vi "IV_Sweep.vi"(8 "error in":errorcluster, 11 "Transport":refnum<class "Transport.lvclass">) -> (0 "error out":errorcluster, 3 "Transport out":refnum<class "Transport.lvclass">)   [LabVIEW 2016, in "Transport.lvclass"]
uses:
  Transport.lvclass
  Control Experiment/Typedefs/Instruments--cluster.ctl
  <userlib>/LevyLab/Krohn Hite 7008/Instrument.KH7008.lvclass
  <userlib>/LevyLab/Lockin-Multichannel/Instrument.Lockin/Instrument.Lockin.lvclass
  <userlib>/LevyLab/Levylab Instruments/Instrument Types/Cryostat/Instrument.Cryostat.lvclass
  <userlib>/LevyLab/Levylab Instruments/Instrument Types/CBridge/Instrument.CBridge.lvclass
  <userlib>/LevyLab/Levylab Instruments/Instrument Types/Optical Delay Line/Instrument.OpticalDelayLine.lvclass
  <userlib>/LevyLab/Levylab Instruments/Instrument Types/Strain/Instrument.Strain.lvclass
  <userlib>/LevyLab/Levylab Instruments/Instrument Types/VNA/Instrument.VNA.lvclass
  <userlib>/LevyLab/Levylab Instruments/Instrument Types/VSource/Instrument.VSource.lvclass
  <userlib>/LevyLab/Lockin-Multichannel/LockinDAQ/Typedefs/AO-cluster.ctl
  <userlib>/LevyLab/Lockin-Multichannel/LockinDAQ/Typedefs/Function-enum.ctl
  <userlib>/LevyLab/Lockin-Multichannel/LockinDAQ/Typedefs/PublicEvents--LockinDAQ.getIVSweepResults.ctl
  Transport.lvclass/Transport.ctl
  Control Experiment/Control Experiment.lvclass/Control Experiment.ctl
  <userlib>/LevyLab/Lockin-Multichannel/LockinDAQ/Typedefs/Sweep Configuration--Cluster.ctl
  Control Experiment/Control Experiment.lvclass
  <userlib>/LevyLab/Lockin-Multichannel/LockinDAQ/LockinDAQ.lvclass
panel:
  out "4Term":cluster{dbl[], dbl[]}[](graph)
  out "2Term":T1(graph)
  in  "Tab Control":T2(tab)
  in  "Sweep IV Step (V)":dbl format="%#_6p"
  in  "Return to Start":bool
  in  "Sweep End (V)":dbl[](array[numeric]) format="%#_6p"
  in  "Sweep Start (V)":dbl[](array[numeric]) format="%#_6p"
  in  "Sweep Channel":i32[](array[numeric])
  in  "OK":bool
  in  "decimating factor":i32=1
  in  "low cutoff freq: fl":dbl=0.01 format="%0.4f"
  out "Temp (K)":dbl
  in  "offset":dbl[](array[numeric])=[0.0, 0.0, 0.0, 0.0, 0.0, 0.0, 0.0, 0.0] format="%_6p"
  in  "invert":dbl[](array[numeric])=[1.0, 1.0, 1.0, 1.0, 1.0, 1.0, 1.0, 1.0] format="%#_6p"
  out "DC Voltages":dbl[](array[numeric])=[0.00025, 0.3, 0.0, 0.0, 0.0, 0.0, 0.0, 0.0, 0.00025, 0.3, 0.0, 0.0, 0.0, 0.0, 0.0, 0.0, 0.00025, 0.3, 0.0, 0.0, 0.0, 0.0, 0.0, 0.0, 0.00025, 0.3, 0.0, 0.0, 0.0, 0.0, 0.0, 0.0, 0.00025, 0.3, 0.0, 0.0, 0.0, 0.0, 0.0, 0.0, 0.00025, 0.3, 0.0, 0.0, 0.0, 0.0, 0.0, 0.0, 0.00025, 0.3, 0.0, 0.0, 0.0, 0.0, 0.0, 0.0, 0.00025, 0.3, 0.0, 0.0, 0.0, 0.0, 0.0, 0.0]
  out "Field (T)":dbl
  in  "Enable Filter?":bool
  in  "Experiment Folder":string="6H_IVcurves"
  in  "Experiment Comments":string="SA03036H\nsweep Vsg:-150mV to 600mV, 1mV steps\nB: 7T to -7T\nVbg = -3.9V\nT: 50mK\n\nlockin\n\nI+/-: 2/3 3mV ac+ 250uV dc bias, 0.4 Hz\nV1+/-: 8/4\nV2+/- 6/28\nV3+/V3-: 27/8\nVsg: 1\nVbg :26\n\ntc 300ms order 2"
  out "time to write files (ms)":u32
  out "sweep time (ms)":u32
  out "total time (ms)":u32
  out "AI Waveform":waveform(dbl)[](graph)
  out "AO Waveform":waveform(dbl)[](graph)
  # "*** These controls are only read if this VI is the top level. If is is called from Sweep Control then the folder and comments come from Sweep Control.vi ***"
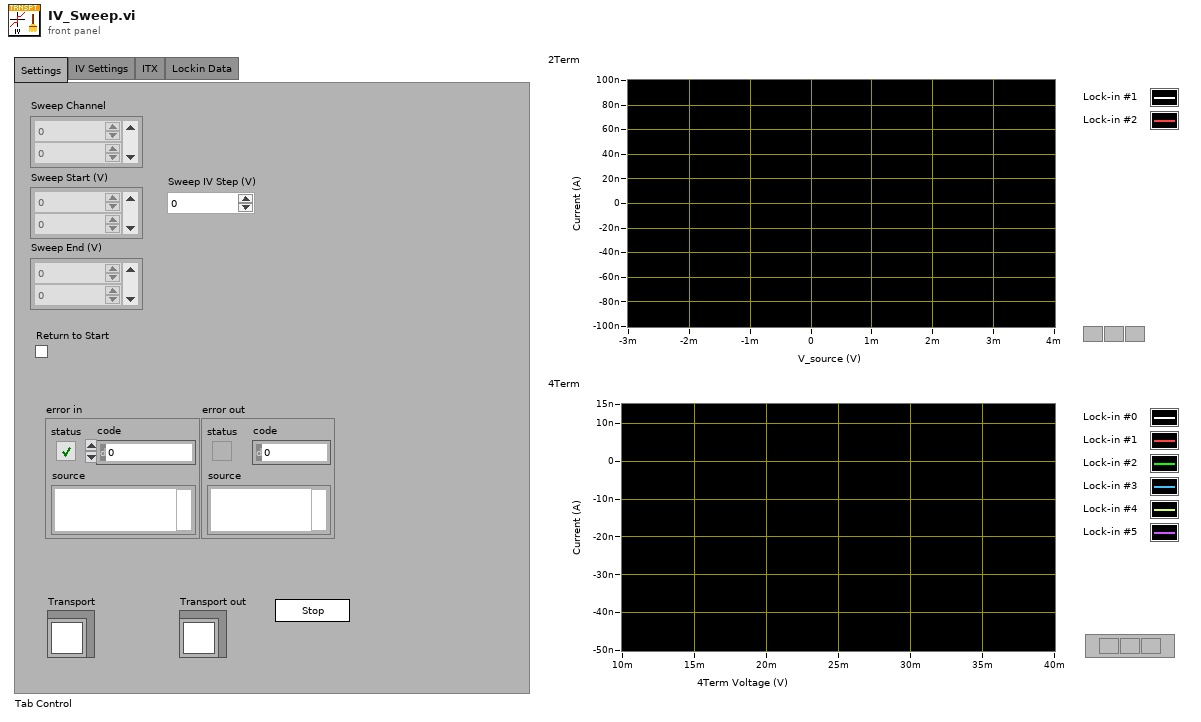
[diagram p1: front panel]
types:
  T1 = cluster{"Decimated and Filtered Array":dbl[], "Decimated and Filtered Array":dbl[]}[]
  T2 = enum32{"Settings", "IV Settings", "ITX", "Lockin Data"}
  T3 = enum32{"Invalid", "Standard", "Closed", "Hidden", "Minimized", "Maximized"}
  T4 = enum32{"invalid app kind", "Development System", "Run Time System", "Student Edition", "Embedded LabVIEW", "Evaluation", "Custom"}
  T5 = typedef "LockinDAQ.lvclass/Sweep Configuration--Cluster.ctl" = cluster{"Sweep Type":enum16{"sweepLockin", "sweepIV"}, "Sweep Lockin Time (s)":dbl, "Sweep IV Step (V)":dbl, "Initial Wait Time (s)":dbl, "Sweep Channel":i32[], "Sweep Start (V)":dbl[], "Sweep End (V)":dbl[], "Return to Start":bool}
  T6 = typedef "Control Experiment.lvclass/Instruments--cluster.ctl" = cluster{"KH7008":refnum<class "Instrument.KH7008.lvclass">[], "Lockin":refnum<class "Instrument.Lockin.lvclass">, "Temperature":refnum<class "Instrument.Cryostat.lvclass">, "Magnet":refnum<class "Instrument.Cryostat.lvclass">, "Rotator":refnum<class "Instrument.Cryostat.lvclass">, "Level":refnum<class "Instrument.Cryostat.lvclass">, "Capacitance Bridge":refnum<class "Instrument.CBridge.lvclass">, "Optical Delay Line":refnum<class "Instrument.OpticalDelayLine.lvclass">, "Strain Cell":refnum<class "Instrument.Strain.lvclass">, "VNA":refnum<class "Instrument.VNA.lvclass">, "Voltage Source":refnum<class "Instrument.VSource.lvclass">}
  T7 = typedef "LockinDAQ.lvclass/AO-cluster.ctl" = cluster{"Ch":i32[], "Amp (V)":dbl[], "DC (V)":dbl[], "f (Hz)":dbl[], "Phase (°)":dbl[], "Function":T8[], "Sweep?":bool[]}
  T8 = typedef "LockinDAQ.lvclass/Function-enum.ctl" = enum16{"Sine", "Triangle", "Square", "Sawtooth"}
  T9 = typedef "LockinDAQ.lvclass/PublicEvents--LockinDAQ.getIVSweepResults.ctl" = cluster{"IVSweepResults []":cluster{"AO":waveform(dbl)[], "AI":waveform(dbl)[]}[], "Sweeping":bool[]}
  T10 = cluster{"Core":cluster{"Current VI Reference":refnum<vi>, "Close Panel on Exit?":bool}, "Transport":refnum<class "Transport.lvclass">, "SweepControl":refnum<class "SweepControl.lvclass">, "Control Experiment":refnum<class "Control Experiment.lvclass">, "Instruments":T6, "Temperature":dbl, "Magnet":dbl, "AOconfig":T7, "getIVSweepResults":T9, "IVSweepResults (filtered)":T9, "Execution:State":enum32{"Bad", "Idle", "Run top level", "Running"}}
  T11 = enum32{"Bad", "Idle", "Run top level", "Running"}
  T12 = cluster{"Current VI Reference":refnum<vi>, "Close Panel on Exit?":bool}
  T13 = cluster{"I-":i32, "I+":i32, "V1-":i32, "V1+":i32, "I2-":i32, "I2+":i32, "V2-":i32, "V2+":i32}
  T14 = cluster{"AO":waveform(dbl)[], "AI":waveform(dbl)[]}[]
  T15 = cluster{"AO":waveform(dbl)[], "AI":waveform(dbl)[]}
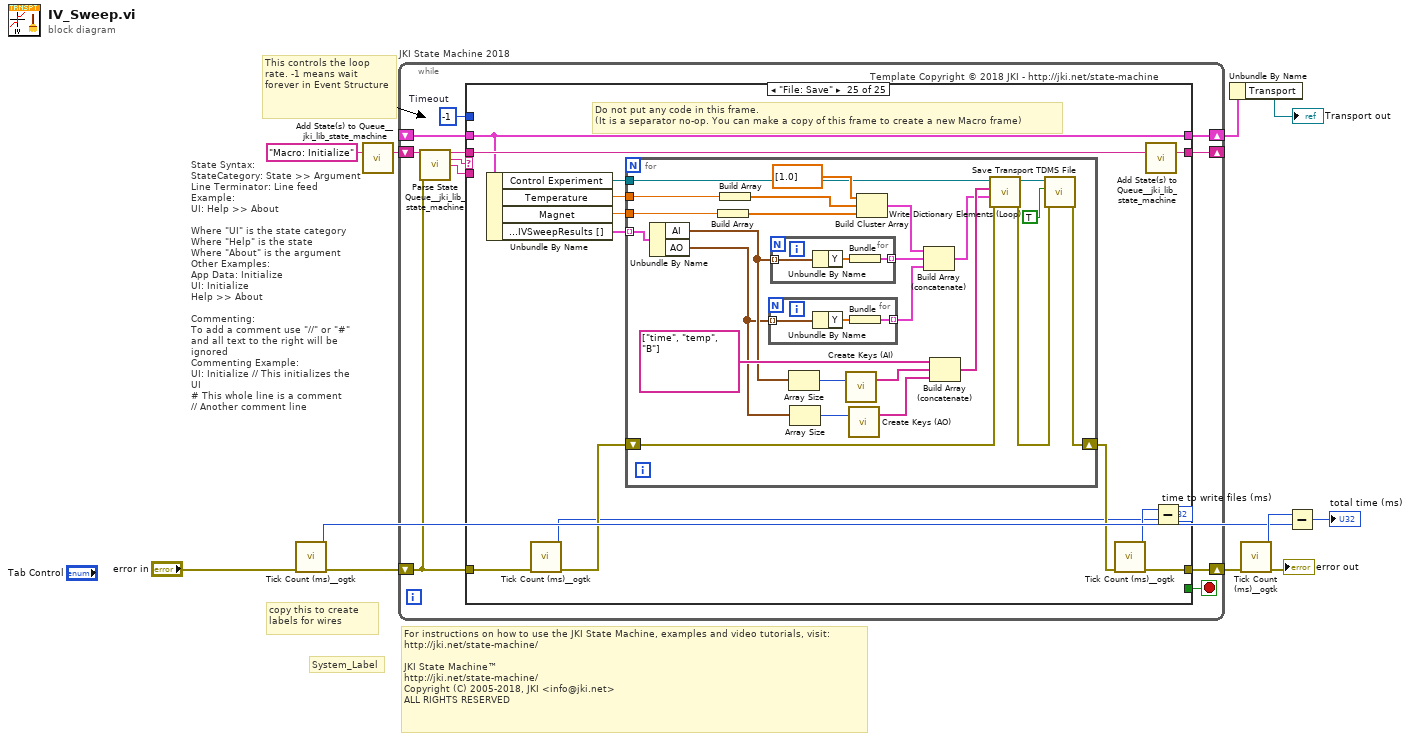
[diagram p0: block diagram]
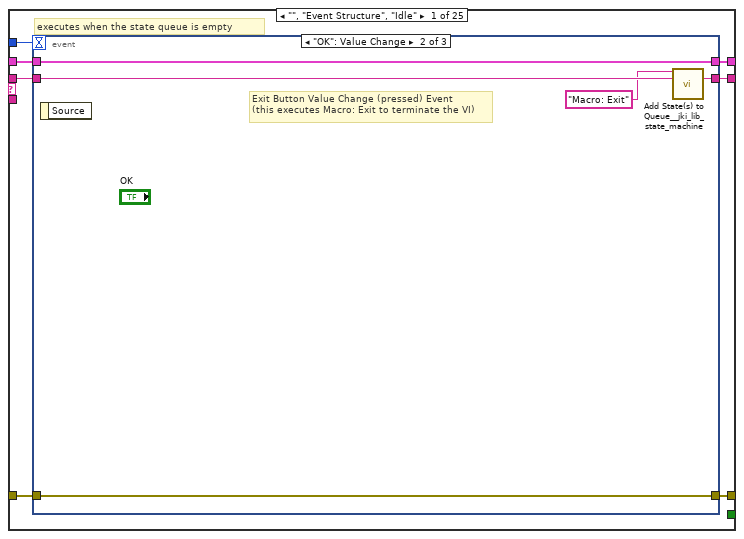
[diagram p2: hidden frame]
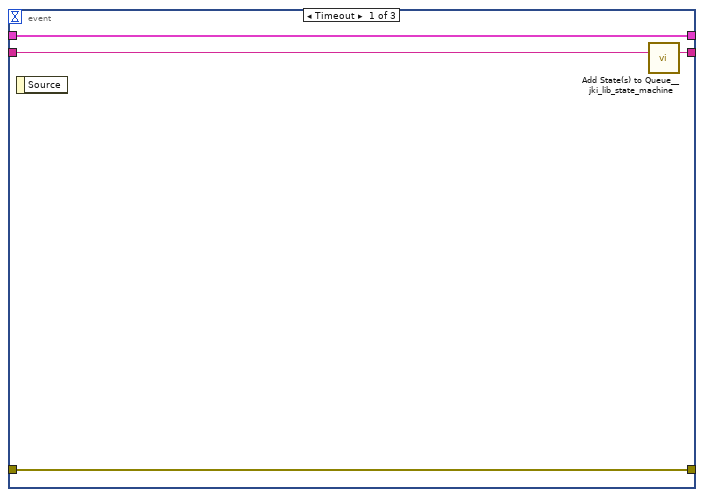
[diagram p3: hidden frame]
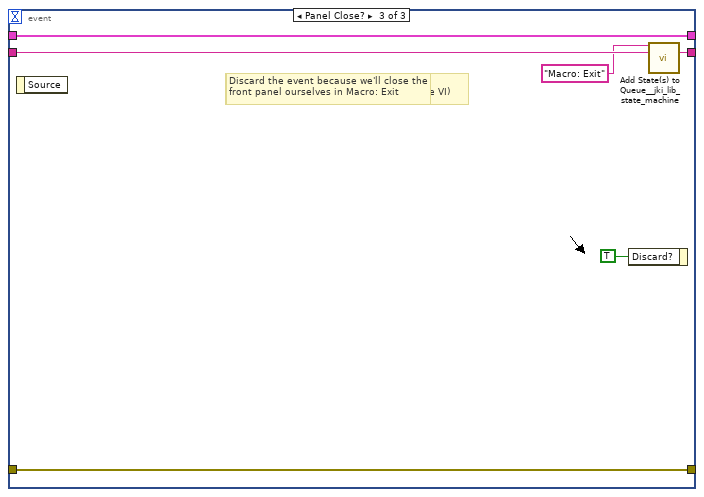
[diagram p4: hidden frame]
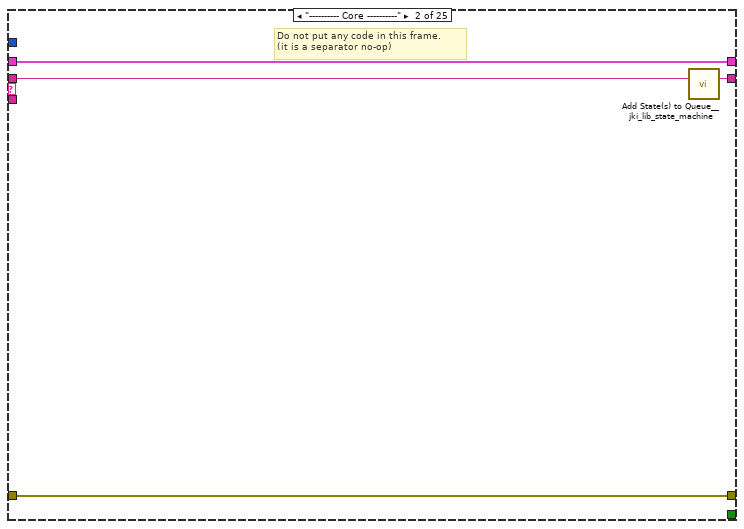
[diagram p5: hidden frame]
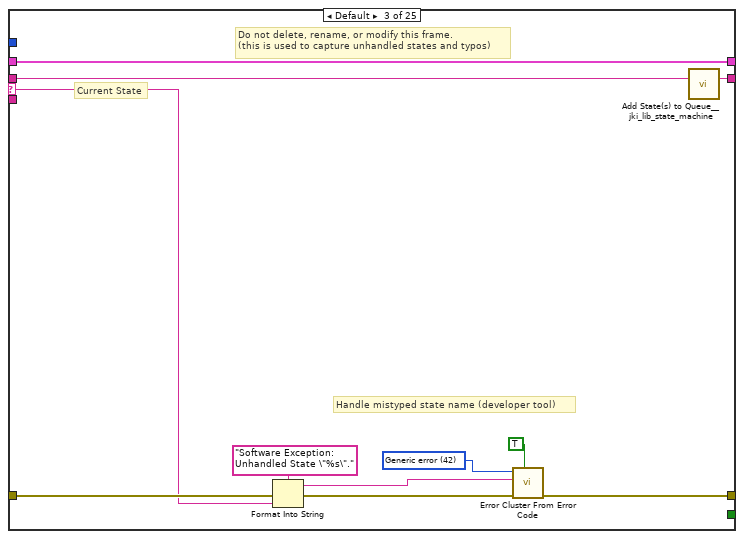
[diagram p6: hidden frame]
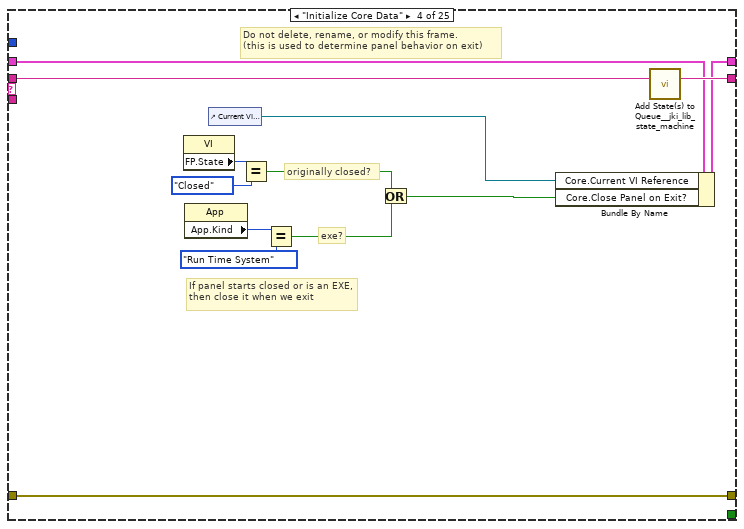
[diagram p7: hidden frame]
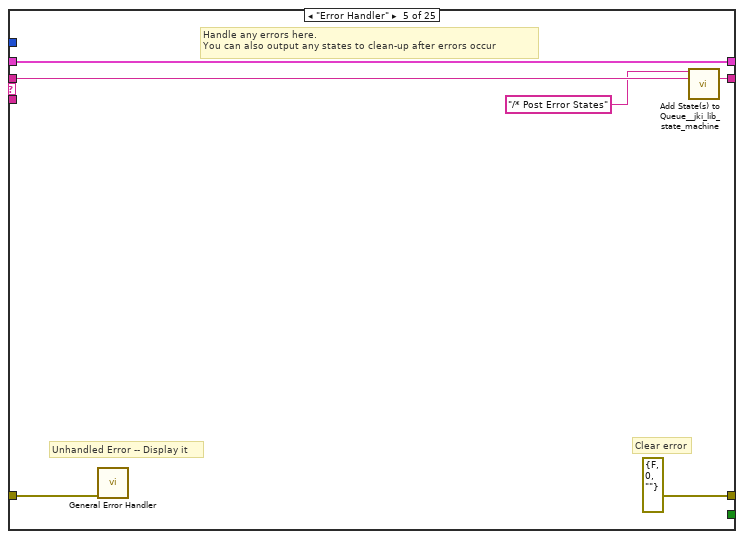
[diagram p8: hidden frame]
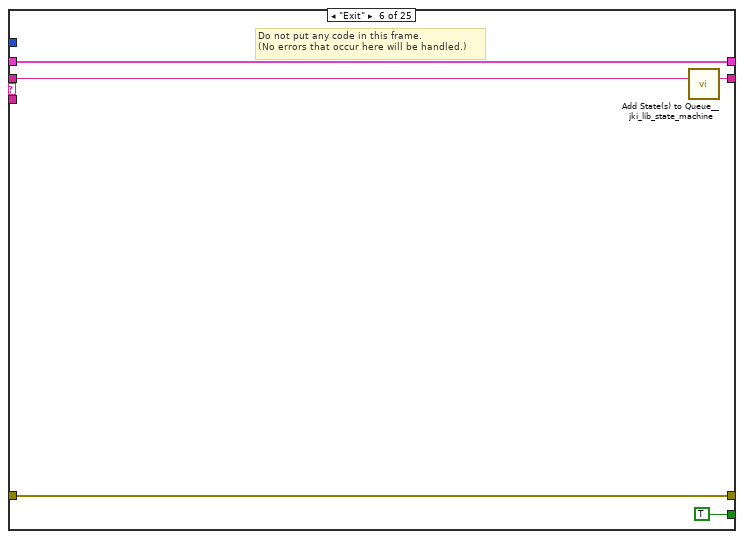
[diagram p9: hidden frame]
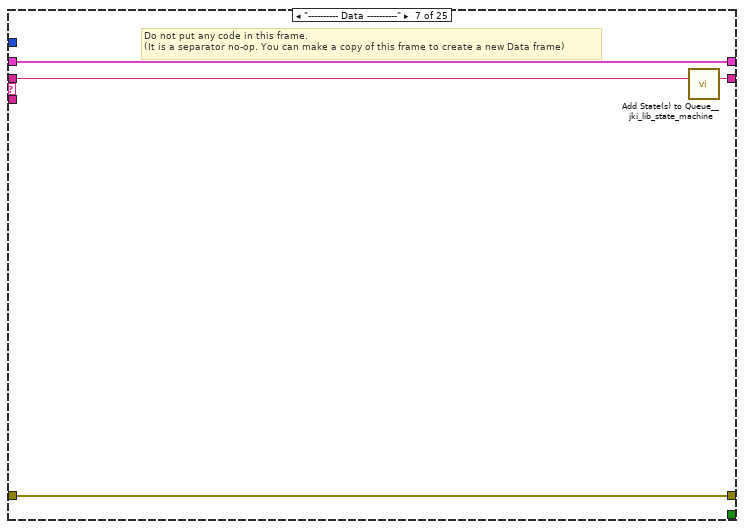
[diagram p10: hidden frame]
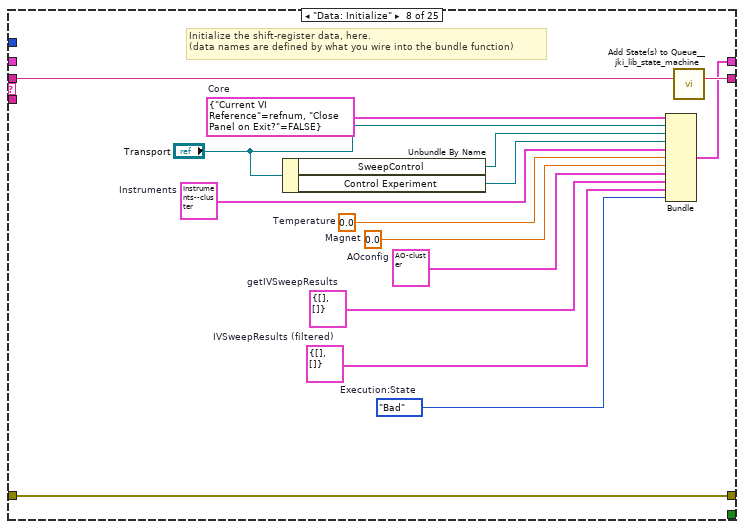
[diagram p11: hidden frame]
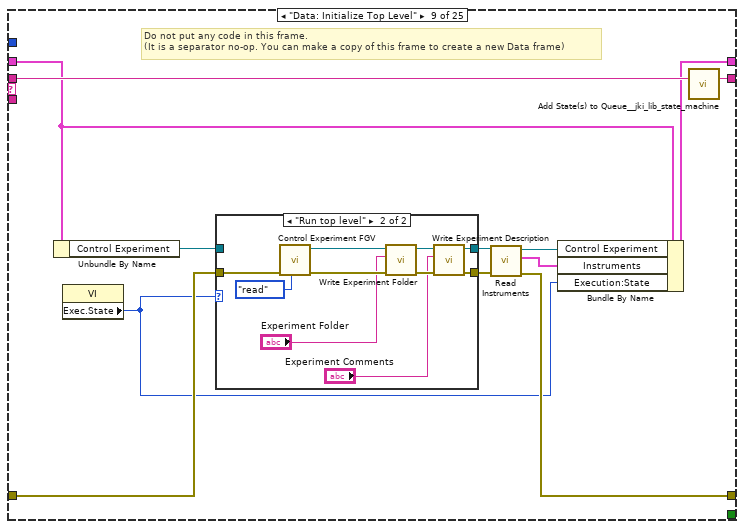
[diagram p12: hidden frame]
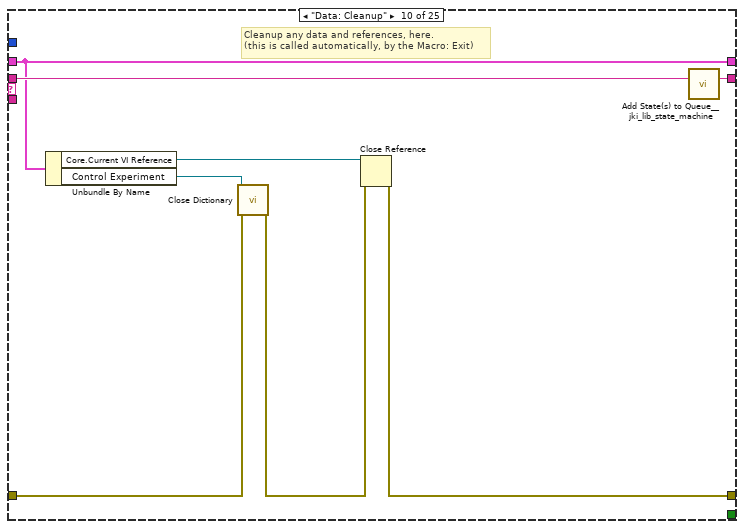
[diagram p14: hidden frame]
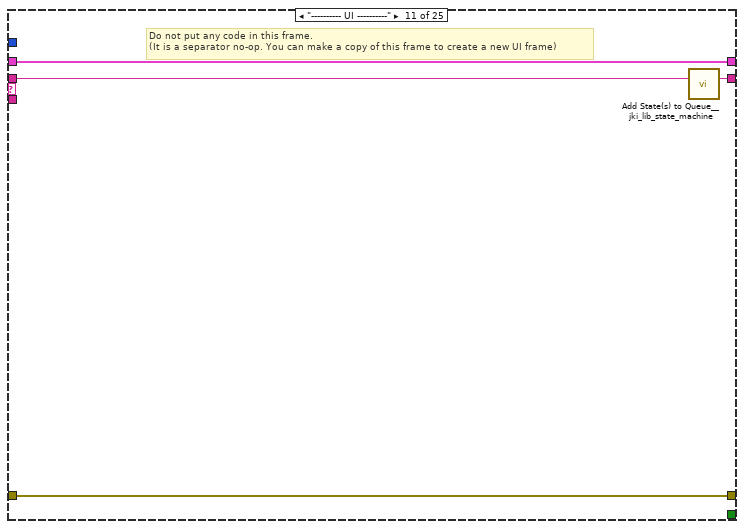
[diagram p15: hidden frame]
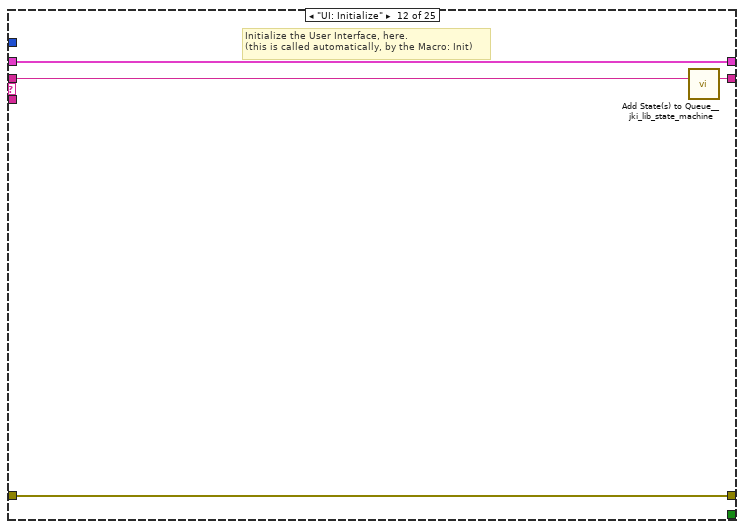
[diagram p16: hidden frame]
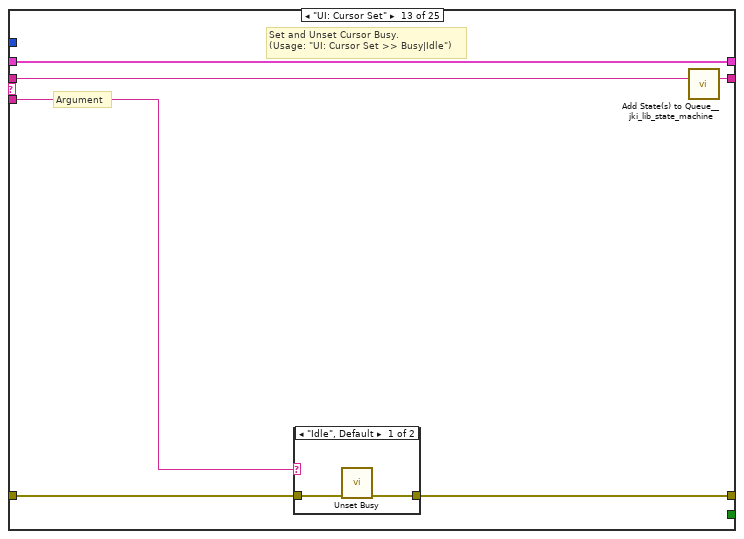
[diagram p17: hidden frame]
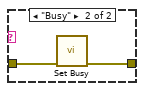
[diagram p18: hidden frame]
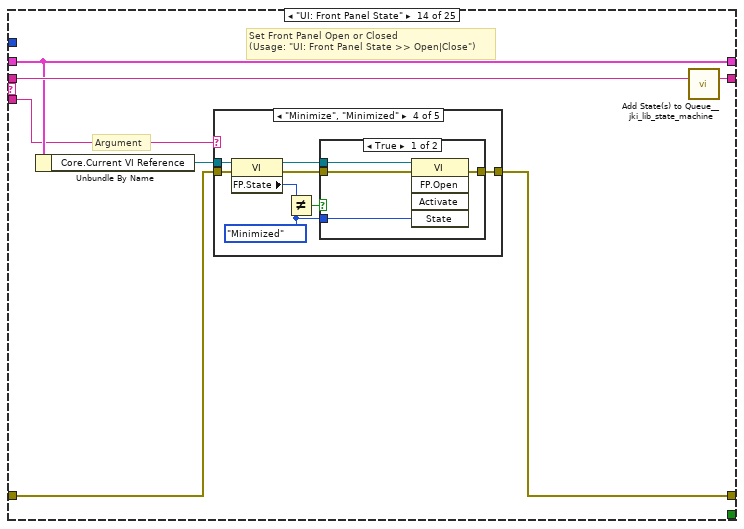
[diagram p19: hidden frame]
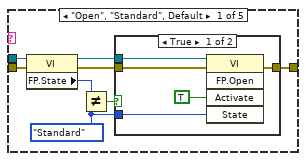
[diagram p20: hidden frame]
diagram:
  # "For instructions on how to use the JKI State Machine, examples and video tutorials, visit:\nhttp://jki.net/state-machine/\n\nJKI State Machine™\nhttp://jki.net/state-machine/\nCopyright (C) 2005-2018, JKI <info@jki.net>\nALL RIGHTS RESERVED"
  # "State Syntax:\nStateCategory: State >> Argument\nLine Terminator: Line feed\nExample:\nUI: Help >> About\n\nWhere \"UI\" is the state category\nWhere \"Help\" is the state\nWhere \"About\" is the argument\nOther Examples:\nApp Data: Initialize\nUI: Initialize\nHelp >> About\n\nCommenting:\nTo add a comment use \"//\" or \"#\" and all text to the right will be ignored\nCommenting Example:\nUI: Initialize // This initializes the UI\n# This whole line is a comment\n// Another comment line"
  # "copy this to create labels for wires"
  # "This controls the loop rate. -1 means wait forever in Event Structure"
  # "System_Label"
  n1 = call <userlib>:"Tick Count (ms)__ogtk.vi"("error in (no error)"="error in") -> ("error out"=w4:errorcluster, "millisecond timer value"=w2:u32)  [unwired: 9 in]
  n2 = call <vilib>:"Add State(s) to Queue__jki_lib_state_machine.vi"("State(s) in (\"\")"="Macro: Initialize") -> ("States Out"=w11:string)  [unwired: 14 in]
  n3 = while "JKI State Machine 2018" {
    shift-right: [w15] -> w9
    shift-left: _ -> [w14]
    shift-right: [w18] -> w6
    shift-left: w4 -> [w12]
    shift-right: [w17] -> _
    shift-left: w11 -> [w19]
    stop <- w16 stop-if-true
    w13 = -1  # Timeout
    # "Template Copyright © 2018 JKI - http://jki.net/state-machine"
    n4 = call <vilib>:"Parse State Queue__jki_lib_state_machine.vi"("State Queue"=w19, "Error In (no error)"=w12) -> ("Remaining States"=w21:string, "Current State"=w22:string, "Arguments"=w20:string)  [unwired: 11 in]
    n5 = case shown="\"File: Save\"" w22 {
      selector: w22 -> [_ _ w49 _ _ _ _ _ _ _ _ _ _ _ _ _ _ _ _ _ _ _ _ _ _]
      tunnel: w21 -> [w29 w48 w53 w72 w78 w83 w87 w102 w114 w134 w138 w142 w148 w159 w228 w237 w271 w276 w286 w290 w303 w323 w330 w363 w377]
      tunnel: w20 -> [_ _ _ _ _ _ _ _ _ _ _ _ w143 w153 _ _ _ _ _ _ _ _ _ _ _]
      tunnel: w14 -> [w27 w45 w51 w65 w75 w81 w84 _ w106 w130 w135 w140 w146 w155 w225 w235 w268 w273 w283 w287 w295 w321 w326 w360 w375]
      tunnel: [w26 w46 w55 w69 errorcluster {"status"=FALSE, "code"=0, "source"=""} ("error out") w80 w85 w99 w107 w131 w136 w139 w144 w156 w226 w233 w269 w274 w284 w288 w292 w307 w328 w361 w367] -> w18
      tunnel: w12 -> [w25 w46 w54 w69 w74 w80 w85 w99 w108 w128 w136 w139 w145 w157 w226 w234 w269 w274 w284 w288 w298 w318 w328 w361 w370]
      tunnel: [w28 w47 w52 w71 w77 w82 w86 w101 w113 w133 w137 w141 w147 w158 w227 w236 w270 w275 w285 w289 w302 w322 w329 w362 w376] -> w17
      tunnel: [_ _ _ _ _ TRUE _ _ _ _ _ _ _ _ _ _ _ _ _ _ _ _ _ _ _] -> w16
      tunnel: [w24 w45 w51 w70 w75 w81 w84 w100 w105 w130 w135 w140 w146 w155 w225 w235 w268 w273 w283 w287 w294 w320 w325 w360 w375] -> w15
      tunnel: w13 -> [w23 _ _ _ _ _ _ _ _ _ _ _ _ _ _ _ _ _ _ _ _ _ _ _ _]
      frame "", "Event Structure", "Idle" {
        # "executes when the state queue is empty"
        n6 = event shown="[1] \"OK\": Value Change" {
          selector: _ -> [_ _ _]
          dyn-events: _ -> [_ _ _]
          timeout: w23 -> [_ _ _]
          tunnel: w29 -> [w33 w38 w44]
          tunnel: [w32 w37 w43] -> w28
          tunnel: w27 -> [w30 w35 w41]
          tunnel: [w31 w36 w42] -> w26
          tunnel: w25 -> [w31 w36 w42]
          tunnel: [w30 w35 w41] -> w24
          event Timeout {
            n7 = event-data() -> ()  [unwired: 1 in, 1 out]
            n8 = call <vilib>:"Add State(s) to Queue__jki_lib_state_machine.vi"("State(s) in (\"\")"=w33) -> ("States Out"=w32:string)  [unwired: 14 in]
          }
          event "OK": Value Change {
            # "Exit Button Value Change (pressed) Event\n(this executes Macro: Exit to terminate the VI)"
            n9 = event-data() -> ()  [unwired: 1 in, 1 out]
            n10 = call <vilib>:"Add State(s) to Queue__jki_lib_state_machine.vi"("State(s) in Front (\"\")"="Macro: Exit", "State(s) in (\"\")"=w38) -> ("States Out"=w37:string)  [unwired: 13 in]
          }
          event Panel Close? {
            # "Discard the event because we'll close the front panel ourselves in Macro: Exit"
            # "Close Panel button (pressed) Event\n(this executes Macro: Exit to terminate the VI)"
            n11 = event-data() -> ()  [unwired: 1 in, 1 out]
            n12 = event-data("Discard?"=TRUE) -> ()  [unwired: 1 in, 1 out]
            n13 = call <vilib>:"Add State(s) to Queue__jki_lib_state_machine.vi"("State(s) in Front (\"\")"="Macro: Exit", "State(s) in (\"\")"=w44) -> ("States Out"=w43:string)  [unwired: 13 in]
          }
        }
      }
      frame "---------- Core ----------" {
        # "Do not put any code in this frame.\n(it is a separator no-op)"
        n14 = call <vilib>:"Add State(s) to Queue__jki_lib_state_machine.vi"("State(s) in (\"\")"=w48) -> ("States Out"=w47:string)  [unwired: 14 in]
      }
      frame Default {
        w58 = 42 items=["No error", "Argument error", "Memory is full", "Out of zone", "End of file", "File already open", "Generic file I/O error", "File not found", "File permission error", "Disk is full", "Duplicate path", "Too many files open", "System feature not enabled", "Resource file not found", "Cannot add resource", "Resource not found", "Image not found", "Image memory error", "Pen does not exist", "Config type invalid", "Config token not found", "Config parse error", "Config memory error", "Bad external code format", "Bad external code offset", "External code not present", "Null window", "Destroy window error", "Null menu", "Print aborted", "Bad print record", "Print driver error", "Windows error during printing", "Memory error during printing", "Print dialog error", "Generic print error", "Invalid device refnum", "Device not found", "Device parameter error", "Device unit error", "Cannot open device", "Device call aborted", "Generic error", "Cancelled by user", "Object ID too low", "Object ID too high", "Object not in heap", "Unknown heap", "Unknown object (invalid DefProc)", "Unknown object (DefProc not in table)", "Message out of range", "Invalid (null) method", "Unknown message", "Manager call not supported", "Bad address", "Network operation in progress", "Network operation timed out", "Connection is busy", "Network attribute not supported", "Network error", "Address in use", "System out of memory", "Connection aborted", "Connection refused", "Not connected", "Already connected", "Connection closed", "Initialization error (interapplication manager)", "Bad occurrence", "Wait on unbound occurrence handler", "Occurrence queue overflow", "Datalog type conflict", "Unused", "Unrecognized type (interapplication manager)", "Memory corrupt", "Failed to make temporary DLL", "Old CIN version", "Drag socket not found", "Failed to load drop-object", "Failed to register OLE object", "Failed to release OLE object", "Format specifier type mismatch", "Unknown format specifier", "Too few format specifiers", "Too many format specifiers", "Scan failed", "Newer CIN version", "Error converting to variant", "Runtime menu error", "Password tampered", "Variant attribute not found", "Incompatible variant data type", "Event data is not available", "Event Store is not present", "Occurrence is not found", "Event Queue is not created", "Event info is not available", "Refnum passed is NULL", "Error retrieving Class GUID", "Error retrieving CoClass GUID", "Error retrieving TypeLib GUID.", "Bad built application magic bytes.", "Specific driver is different from the specific driver associated with the Logical Name.", "There is no session opened to the class driver.", "Max Error", "MAX - Error with config objects", "MAX - Error loading configuration", "MAX - Group not supported"]
        # "Current State"
        # "Do not delete, rename, or modify this frame.\n(this is used to capture unhandled states and typos)"
        # "Handle mistyped state name (developer tool)"
        n15 = Format Into String(format string="Software Exception: Unhandled State \"%s\"." ("message"), error in=w54, w49) -> (resulting string=w57:string, error out=w56:errorcluster)  [unwired: 1 in]
        n16 = call <vilib>:"Error Cluster From Error Code.vi"("show call chain? (False)"=TRUE, "error in (no error)"=w56, "error message (\"\")"=w57, "error code (0)"=w58) -> ("error out"=w55:errorcluster)  [unwired: 5 in]
        n17 = call <vilib>:"Add State(s) to Queue__jki_lib_state_machine.vi"("State(s) in (\"\")"=w53) -> ("States Out"=w52:string)  [unwired: 14 in]
      }
      frame "Initialize Core Data" {
        # "Do not delete, rename, or modify this frame.\n(this is used to determine panel behavior on exit)"
        # "originally closed?"
        # "exe?"
        # "If panel starts closed or is an EXE, then close it when we exit"
        n18 = property class="VI"() -> ("FP.State"=w62:T3)  [unwired: 2 in, 2 out]
        n19 = property class="App"() -> ("App.Kind"=w68:T4)  [unwired: 2 in, 2 out]
        n20 = control-ref of="Current VI Reference"() -> (w63:refnum<vi>)
        n21 = Equal?(x=w62, y=T3."Closed" ("Front Panel Window:State")) -> (x = y?=w60:bool)
        n22 = Equal?(x=w68, y=T4."Run Time System" ("Application:Kind")) -> (x = y?=w66:bool)
        n23 = Or(x=w60, y=w66) -> (x .or. y?=w64:bool)
        n24 = Bundle By Name(cluster=w65, "Core.Current VI Reference"=w63, "Core.Close Panel on Exit?"=w64) -> (w70:T10)
        n25 = call <vilib>:"Add State(s) to Queue__jki_lib_state_machine.vi"("State(s) in (\"\")"=w72) -> ("States Out"=w71:string)  [unwired: 14 in]
      }
      frame "Error Handler" {
        # "Unhandled Error -- Display it"
        # "Handle any errors here.\nYou can also output any states to clean-up after errors occur"
        # "Clear error"
        n26 = call <vilib>:"General Error Handler.vi"("error in (no error)"=w74) -> ()  [unwired: 10 in, 5 out]
        n27 = call <vilib>:"Add State(s) to Queue__jki_lib_state_machine.vi"("State(s) in Front (\"\")"="/* Post Error States", "State(s) in (\"\")"=w78) -> ("States Out"=w77:string)  [unwired: 13 in]
      }
      frame "Exit" {
        # "Do not put any code in this frame.\n(No errors that occur here will be handled.)"
        n28 = call <vilib>:"Add State(s) to Queue__jki_lib_state_machine.vi"("State(s) in (\"\")"=w83) -> ("States Out"=w82:string)  [unwired: 14 in]
      }
      frame "---------- Data ----------" {
        # "Do not put any code in this frame.\n(It is a separator no-op. You can make a copy of this frame to create a new Data frame)"
        n29 = call <vilib>:"Add State(s) to Queue__jki_lib_state_machine.vi"("State(s) in (\"\")"=w87) -> ("States Out"=w86:string)  [unwired: 14 in]
      }
      frame "Data: Initialize" {
        w88 = T11."Bad"  # Execution:State
        w89 = T9 {"IVSweepResults []"=[], "Sweeping"=[]}  # IVSweepResults (filtered)
        w90 = T9 {"IVSweepResults []"=[], "Sweeping"=[]}  # getIVSweepResults
        w91 = 0.0  # Magnet
        w92 = 0.0  # Temperature
        w93 = T7 {"Ch"=[], "Amp (V)"=[0.01, 0.0, 0.0, 0.0, 0.0, 0.0, 0.0, 0.0], "DC (V)"=[0.0, 0.0, 0.0, 0.0, 0.0, 0.0, 0.0, 0.0], "f (Hz)"=[0.0, 0.0, 0.0, 0.0, 0.0, 0.0, 0.0, 0.0], "Phase (°)"=[13.1, 13.0, 13.0, 13.0, 13.0, 13.0, 13.0, 13.0], "Function"=[enum."Sine", enum."Sine", enum."Sine", enum."Sine", enum."Sine", enum."Sine", enum."Sine", enum."Sine"], "Sweep?"=[]}  # AOconfig
        w94 = T6 {"KH7008"=[], "Lockin"=refnum, "Temperature"=refnum, "Magnet"=refnum, "Rotator"=refnum, "Level"=refnum, "Capacitance Bridge"=refnum, "Optical Delay Line"=refnum, "Strain Cell"=refnum, "VNA"=refnum, "Voltage Source"=refnum}  # Instruments
        w98 = T12 {"Current VI Reference"=refnum, "Close Panel on Exit?"=FALSE}  # Core
        # "Initialize the shift-register data, here.\n(data names are defined by what you wire into the bundle function)"
        n30 = Unbundle By Name("Transport") -> ("SweepControl"=w96:refnum<class "SweepControl.lvclass">, "Control Experiment"=w95:refnum<class "Control Experiment.lvclass">)
        n31 = Bundle("Core"=w98, "Transport"="Transport", "SweepControl"=w96, "Control Experiment"=w95, "Instruments"=w94, "Temperature"=w92, "Magnet"=w91, "AOconfig"=w93, "getIVSweepResults"=w90, "IVSweepResults (filtered)"=w89, "Execution:State"=w88) -> (w100:T10)  [unwired: 1 in]
        n32 = call <vilib>:"Add State(s) to Queue__jki_lib_state_machine.vi"("State(s) in (\"\")"=w102) -> ("States Out"=w101:string)  [unwired: 14 in]
      }
      frame "Data: Initialize Top Level" {
        # "Do not put any code in this frame.\n(It is a separator no-op. You can make a copy of this frame to create a new Data frame)"
        n33 = Unbundle By Name(w106) -> ("Control Experiment"=w104:refnum<class "Control Experiment.lvclass">)
        n34 = property class="VI"() -> ("Exec.State"=w103:T11)  [unwired: 2 in, 2 out]
        n35 = case shown="\"Run top level\"" w103 {
          tunnel: [w115 w122] -> w110
          tunnel: [w116 w121] -> w109
          tunnel: w108 -> [w115 w120]
          tunnel: w104 -> [w116 _]
          frame Default {
          }
          frame "Run top level" {
            n36 = call "Control Experiment FGV.vi"("Function"=enum16{"read", "write"}."read", "error in (no error)"=w120) -> ("error out"=w125:errorcluster, "Control Experiment.lvclass out"=w126:refnum<class "Control Experiment.lvclass">)  [unwired: 8 in]
            n37 = call "Write Experiment Folder.vi"("error in (no error)"=w125, "Experiment Folder"="Experiment Folder", "Control Experiment in"=w126) -> ("error out"=w123:errorcluster, "Control Experiment out"=w124:refnum<class "Control Experiment.lvclass">)  [unwired: 7 in]
            n38 = call "Write Experiment Description.vi"("error in (no error)"=w123, "Experiment Description"="Experiment Comments", "Control Experiment in"=w124) -> ("error out"=w122:errorcluster, "Control Experiment out"=w121:refnum<class "Control Experiment.lvclass">)  [unwired: 7 in]
          }
        }
        n39 = call "Read Instruments.vi"("error in (no error)"=w110, "Control Experiment in"=w109) -> ("error out"=w107:errorcluster, "Instruments"=w111:T6, "Control Experiment out"=w112:refnum<class "Control Experiment.lvclass">)  [unwired: 7 in]
        n40 = Bundle By Name(cluster=w106, "Control Experiment"=w112, "Instruments"=w111, "Execution:State"=w103) -> (w105:T10)
        n41 = call <vilib>:"Add State(s) to Queue__jki_lib_state_machine.vi"("State(s) in (\"\")"=w114) -> ("States Out"=w113:string)  [unwired: 14 in]
      }
      frame "Data: Cleanup" {
        # "Cleanup any data and references, here.\n(this is called automatically, by the Macro: Exit)"
        n42 = Unbundle By Name(w130) -> ("Core.Current VI Reference"=w132:refnum<vi>, "Control Experiment"=w129:refnum<class "Control Experiment.lvclass">)
        n43 = call "Close Dictionary.vi"("error in (no error)"=w128, "Control Experiment in"=w129) -> ("error out"=w127:errorcluster)  [unwired: 8 in, 1 out]
        n44 = Close Reference(reference=w132, error in (no error)=w127) -> (error out=w131:errorcluster)
        n45 = call <vilib>:"Add State(s) to Queue__jki_lib_state_machine.vi"("State(s) in (\"\")"=w134) -> ("States Out"=w133:string)  [unwired: 14 in]
      }
      frame "---------- UI ----------" {
        # "Do not put any code in this frame.\n(It is a separator no-op. You can make a copy of this frame to create a new UI frame)"
        n46 = call <vilib>:"Add State(s) to Queue__jki_lib_state_machine.vi"("State(s) in (\"\")"=w138) -> ("States Out"=w137:string)  [unwired: 14 in]
      }
      frame "UI: Initialize" {
        # "Initialize the User Interface, here.\n(this is called automatically, by the Macro: Init)"
        n47 = call <vilib>:"Add State(s) to Queue__jki_lib_state_machine.vi"("State(s) in (\"\")"=w142) -> ("States Out"=w141:string)  [unwired: 14 in]
      }
      frame "UI: Cursor Set" {
        # "Argument"
        # "Set and Unset Cursor Busy.\n(Usage: \"UI: Cursor Set >> Busy|Idle\")"
        n48 = case shown="\"Idle\", Default" w143 {
          tunnel: w145 -> [w150 w152]
          tunnel: [w149 w151] -> w144
          frame "Idle", Default {
            n49 = call <vilib>:"Unset Busy.vi"("error in (no error)"=w150) -> ("error out"=w149:errorcluster)  [unwired: 10 in]
          }
          frame "Busy" {
            n50 = call <vilib>:"Set Busy.vi"("error in (no error)"=w152) -> ("error out"=w151:errorcluster)  [unwired: 9 in, 1 out]
          }
        }
        n51 = call <vilib>:"Add State(s) to Queue__jki_lib_state_machine.vi"("State(s) in (\"\")"=w148) -> ("States Out"=w147:string)  [unwired: 14 in]
      }
      frame "UI: Front Panel State" {
        # "Argument"
        # "Set Front Panel Open or Closed\n(Usage: \"UI: Front Panel State >> Open|Close\")"
        n52 = Unbundle By Name(w155) -> ("Core.Current VI Reference"=w154:refnum<vi>)
        n53 = case shown="\"Minimize\", \"Minimized\"" w153 {
          tunnel: w157 -> [w165 w180 w191 w204 w217]
          tunnel: [w167 w181 w193 w206 w219] -> w156
          tunnel: w154 -> [w166 w178 w192 w205 w218]
          frame "Open", "Standard", Default {
            w160 = T3."Standard" ("State")
            n54 = property class="VI"(reference=w166, error in=w165) -> (reference out=w163:refnum<vi>, error out=w164:errorcluster, "FP.State"=w162:T3)
            n55 = Not Equal?(x=w162, y=w160) -> (x != y?=w161:bool)
            n56 = case shown="True" w161 {
              tunnel: [w171 w173] -> w167
              tunnel: w164 -> [w170 w173]
              tunnel: w163 -> [w169 _]
              tunnel: w160 -> [w168 _]
              frame True {
                n57 = invoke class="VI" method="FP.Open"(reference=w169, error in=w170, "Activate"=TRUE, "State"=w168) -> (error out=w171:errorcluster)  [unwired: 1 in, 4 out]
              }
              frame False {
              }
            }
          }
          frame "Close", "Closed" {
            n58 = property class="VI"(reference=w178, error in=w180) -> (reference out=w177:refnum<vi>, error out=w179:errorcluster, "FP.State"=w175:T3)
            n59 = Not Equal?(x=w175, y=T3."Closed" ("Front Panel Window:State")) -> (x != y?=w174:bool)
            n60 = case shown="True" w174 {
              tunnel: [w182 w185] -> w181
              tunnel: w179 -> [w182 w184]
              tunnel: w177 -> [_ w183]
              frame False {
              }
              frame True {
                n61 = invoke class="VI" method="FP.Close"(reference=w183, error in=w184) -> (error out=w185:errorcluster)  [unwired: 1 in, 2 out]
              }
            }
          }
          frame "Hidden", "Hide" {
            w186 = T3."Hidden" ("State")
            n62 = property class="VI"(reference=w192, error in=w191) -> (reference out=w189:refnum<vi>, error out=w190:errorcluster, "FP.State"=w188:T3)
            n63 = Not Equal?(x=w188, y=w186) -> (x != y?=w187:bool)
            n64 = case shown="True" w187 {
              tunnel: [w197 w198] -> w193
              tunnel: w190 -> [w196 w198]
              tunnel: w189 -> [w195 _]
              tunnel: w186 -> [w194 _]
              frame True {
                n65 = invoke class="VI" method="FP.Open"(reference=w195, error in=w196, "State"=w194) -> (error out=w197:errorcluster)  [unwired: 2 in, 4 out]
              }
              frame False {
              }
            }
          }
          frame "Minimize", "Minimized" {
            w199 = T3."Minimized" ("State")
            n66 = property class="VI"(reference=w205, error in=w204) -> (reference out=w202:refnum<vi>, error out=w203:errorcluster, "FP.State"=w201:T3)
            n67 = Not Equal?(x=w201, y=w199) -> (x != y?=w200:bool)
            n68 = case shown="True" w200 {
              tunnel: [w210 w211] -> w206
              tunnel: w203 -> [w209 w211]
              tunnel: w202 -> [w208 _]
              tunnel: w199 -> [w207 _]
              frame True {
                n69 = invoke class="VI" method="FP.Open"(reference=w208, error in=w209, "State"=w207) -> (error out=w210:errorcluster)  [unwired: 2 in, 4 out]
              }
              frame False {
              }
            }
          }
          frame "Maximize", "Maximized" {
            w212 = T3."Maximized" ("State")
            n70 = property class="VI"(reference=w218, error in=w217) -> (reference out=w215:refnum<vi>, error out=w216:errorcluster, "FP.State"=w214:T3)
            n71 = Not Equal?(x=w214, y=w212) -> (x != y?=w213:bool)
            n72 = case shown="True" w213 {
              tunnel: [w223 w224] -> w219
              tunnel: w216 -> [w222 w224]
              tunnel: w215 -> [w221 _]
              tunnel: w212 -> [w220 _]
              frame True {
                n73 = invoke class="VI" method="FP.Open"(reference=w221, error in=w222, "State"=w220) -> (error out=w223:errorcluster)  [unwired: 2 in, 4 out]
              }
              frame False {
              }
            }
          }
        }
        n74 = call <vilib>:"Add State(s) to Queue__jki_lib_state_machine.vi"("State(s) in (\"\")"=w159) -> ("States Out"=w158:string)  [unwired: 14 in]
      }
      frame "UI: Update Input Graphs" {
        # "Do not put any code in this frame.\n(It is a separator no-op. You can make a copy of this frame to create a new UI frame)"
        n75 = disable-structure shown="Disabled" {
          disable-tunnel: w225 -> [w229 _]
          frame Disabled {
            n76 = Unbundle By Name(w229) -> ("AOconfig.DC (V)"=→"DC Voltages":dbl[], "AO Waveforrm"=→"AO Waveform", "AI Waveform"=→"AI Waveform")
          }
          frame Enabled {
          }
        }
        n77 = call <vilib>:"Add State(s) to Queue__jki_lib_state_machine.vi"("State(s) in (\"\")"=w228) -> ("States Out"=w227:string)  [unwired: 14 in]
      }
      frame "UI: Update IV Graphs" {
        # "Do not put any code in this frame.\n(It is a separator no-op. You can make a copy of this frame to create a new UI frame)"
        n78 = disable-structure shown="Enabled" {
          disable-tunnel: w235 -> [w248 _]
          disable-tunnel: w234 -> [w242 w267]
          disable-tunnel: [w241 w267] -> w233
          frame Disabled {
            # "Decimated AO"
            # "Decimataed AI"
            n79 = Unbundle By Name(w248) -> ("AI (filtered)"=w247, "AO (filtered)"=w246, "Control Experiment"=w243:refnum<class "Control Experiment.lvclass">)
            n80 = call "Get Channel Indices.vi"("error in (no error)"=w242, "Control Experiment in"=w243) -> ("error out"=w241:errorcluster, "Indices"=w238:T13)  [unwired: 7 in, 1 out]
            n81 = Unbundle By Name(w238) -> ("I-"=w245:i32, "V1+"=w239:i32, "V1-"=w240:i32, "I+"=w244:i32)
            n82 = Decrement(x=w245) -> (x-1=w251:i32)
            n83 = Decrement(x=w239) -> (x-1=w260:i32)
            n84 = Decrement(x=w240) -> (x-1=w254:i32)
            n85 = Decrement(x=w244) -> (x-1=w263:i32)
            n86 = Index Array(array=w246, index=w263) -> (element=w264)
            n87 = Index Array(array=w247, index #1=w251, index #2=w260, index #3=w254) -> (element #1=w257, element #2=w253, element #3=w259)
            n88 = Equal?(x=w260, y=w254) -> (x = y?=w255:bool)
            n89 = Subtract(x=w253, y=w259) -> (x-y=w252:dbl)
            n90 = Select(t=w253, s=w255, f=w252) -> (s? t:f=w256:dbl)
            n91 = Unbundle(w257) -> (w261)
            n92 = Unbundle(w264) -> (w262)
            n93 = Unbundle(w256) -> (w258)
            n94 = Bundle(w258, w261) -> (w249:cluster{void, void})  [unwired: 1 in]
            n95 = Bundle(w262, w261) -> (w265:cluster{void, void})  [unwired: 1 in]
            n96 = Build Array(w249) -> (→"4Term":cluster{void, void}[])
            n97 = Build Array(w265) -> (→"2Term":cluster{void, void}[])
          }
          frame Enabled {
          }
        }
        n98 = call <vilib>:"Add State(s) to Queue__jki_lib_state_machine.vi"("State(s) in (\"\")"=w237) -> ("States Out"=w236:string)  [unwired: 14 in]
      }
      frame "---------- Macro ----------" {
        # "Do not put any code in this frame.\n(It is a separator no-op. You can make a copy of this frame to create a new Macro frame)"
        n99 = call <vilib>:"Add State(s) to Queue__jki_lib_state_machine.vi"("State(s) in (\"\")"=w271) -> ("States Out"=w270:string)  [unwired: 14 in]
      }
      frame "Macro: Initialize" {
        w272 = "Data: Initialize\nInitialize Core Data\nUI: Initialize\nUI: Front Panel State >> Open\nData: Initialize Top Level\nMeasure: Cryostat\nMeasure: Lockin\nMeasure: Filter and Decimate\nUI: Update Input Graphs\nUI: Update IV Graphs\nFile: Save\nMacro: Exit"  # Data: Initialize Initialize Core Data UI: Initialize UI: Front Panel State >> Open Data: Initialize Top Level Measure: Cryostat Measure: Lockin Measure: Filter and Decimate UI: Update Input Graphs UI: Update IV Graphs File: Save Macro: Exit
        # "Initialization Macro\n(This is called once, when the VI starts)"
        n100 = call <vilib>:"Add State(s) to Queue__jki_lib_state_machine.vi"("State(s) in Front (\"\")"=w272, "State(s) in (\"\")"=w276) -> ("States Out"=w275:string)  [unwired: 13 in]
      }
      frame "Macro: Exit" {
        # "Exit Macro\n(This is called once, when the VI exits)"
        n101 = Unbundle By Name(w283) -> ("Core.Close Panel on Exit?"=w282:bool)
        n102 = Select(t="UI: Front Panel State >> Close", s=w282, f="") -> (s? t:f=w279:string)
        n103 = call <vilib>:"Add State(s) to Queue__jki_lib_state_machine.vi"("State(s) in (\"\")"=w279, "State(s) at Back (\"\")"="Data: Cleanup\nExit") -> ("States Out"=w277:string)  [unwired: 13 in]
        n104 = call <vilib>:"Add State(s) to Queue__jki_lib_state_machine.vi"("State(s) in Front (\"\")"=w277, "State(s) in (\"\")"=w286) -> ("States Out"=w285:string)  [unwired: 13 in]
      }
      frame "---------- Measure ----------" {
        # "Template Separator\n(You can make a copy of, or modify, this frame)"
        n105 = call <vilib>:"Add State(s) to Queue__jki_lib_state_machine.vi"("State(s) in (\"\")"=w290) -> ("States Out"=w289:string)  [unwired: 14 in]
      }
      frame "Measure: Cryostat" {
        # "Your code here.\n(You can make a copy of, or modify, this frame)"
        n106 = Unbundle By Name(w295) -> ("Instruments.Magnet"=w300:refnum<class "Instrument.Cryostat.lvclass">, "Instruments.Temperature"=w299:refnum<class "Instrument.Cryostat.lvclass">)
        n107 = call-dynamic "Get Temperature.vi"("error in (no error)"=w298, "Instrument.Cryostat in"=w299) -> ("error out"=w301:errorcluster, "Temperature (K)"=w296:dbl)  [unwired: 5 in, 3 out]
        "Temp (K)" <- w296
        n108 = call-dynamic "Get Magnet Field.vi"("error in (no error)"=w301, "Instrument.Cryostat in"=w300) -> ("error out"=w293:errorcluster, "B Field (T)"=w297:dbl)  [unwired: 5 in, 3 out]
        "Field (T)" <- w297
        n109 = Bundle By Name(cluster=w295, "Temperature"=w296, "Magnet"=w297) -> (w294:T10)
        n110 = call <vilib>:"Clear Errors.vi"("error in (no error)"=w293, "specific error code to clear (0: all)"=4000) -> ("error out"=w292:errorcluster)  [unwired: 4 in, 1 out]
        n111 = call <vilib>:"Add State(s) to Queue__jki_lib_state_machine.vi"("State(s) in (\"\")"=w303) -> ("States Out"=w302:string)  [unwired: 14 in]
      }
      frame "Measure: Lockin" {
        # "Your code here.\n(You can make a copy of, or modify, this frame)"
        n112 = Unbundle By Name(w321) -> ("Instruments.Lockin"=w319:refnum<class "Instrument.Lockin.lvclass">)
        n113 = call <userlib>:"Tick Count (ms)__ogtk.vi"("error in (no error)"=w318) -> ("error out"=w308:errorcluster, "millisecond timer value"=w305:u32)  [unwired: 9 in]
        n114 = Bundle By Name(cluster=T5 {"Sweep Type"=enum."sweepLockin", "Sweep Lockin Time (s)"=0.0, "Sweep IV Step (V)"=0.0, "Initial Wait Time (s)"=0.0, "Sweep Channel"=[], "Sweep Start (V)"=[], "Sweep End (V)"=[], "Return to Start"=FALSE} ("Configure Sweep"), "Sweep Channel"="Sweep Channel", "Sweep Start (V)"="Sweep Start (V)", "Sweep End (V)"="Sweep End (V)", "Sweep IV Step (V)"="Sweep IV Step (V)", "Return to Start"="Return to Start") -> (w315:T5)
        n115 = call <userlib>:"startIVSweepAndWait.vi"("error in (no error)"=w308, "Configure Sweep"=w315, "Instrument.Lockin in"=w319) -> ("error out"=w317:errorcluster, "getIVSweepResults"=w314:T9)  [unwired: 6 in, 1 out]
        n116 = Bundle By Name(cluster=w321, "getIVSweepResults"=w314) -> (w320:T10)
        n117 = call <userlib>:"Tick Count (ms)__ogtk.vi"("error in (no error)"=w317) -> ("error out"=w307:errorcluster, "millisecond timer value"=w306:u32)  [unwired: 9 in]
        n118 = Subtract(x=w306, y=w305) -> (x-y=→"sweep time (ms)":u32)
        n119 = call <vilib>:"Add State(s) to Queue__jki_lib_state_machine.vi"("State(s) in (\"\")"=w323) -> ("States Out"=w322:string)  [unwired: 14 in]
      }
      frame "Measure: Filter and Decimate" {
        # "Template Separator\n(You can make a copy of, or modify, this frame)"
        n120 = Unbundle By Name(w326) -> ("getIVSweepResults.IVSweepResults []"=w327:T14)
        n121 = for {
          tunnel: w327 -> [w334] mode=indexing
          tunnel: [w331] -> w324 mode=indexing
          # "AI"
          # "AO"
          n122 = Unbundle By Name(w334) -> ("AI"=w336:waveform(dbl)[], "AO"=w335:waveform(dbl)[])
          n123 = for {
            tunnel: w336 -> [w358] mode=indexing
            tunnel: [w359] -> w341 mode=indexing
            tunnel: "offset" -> [w355] mode=indexing
            tunnel: "invert" -> [w357] mode=indexing
            n124 = Multiply(x=w358, y=w357) -> (x*y=w356:waveform(dbl))
            n125 = Add(x=w356, y=w355) -> (x+y=w359:waveform(dbl))
          }
          n126 = for {
            tunnel: "low cutoff freq: fl" -> [w347]
            tunnel: w335 -> [w344] mode=indexing
            tunnel: "decimating factor" -> [w348]
            tunnel: "Enable Filter?" -> [w346]
            tunnel: [w343] -> w332 mode=indexing
            n127 = call "Decimate and Filter.vi"("Enabled?"=w346, "low cutoff freq: fl"=w347, "decimating factor"=w348, "Waveform in"=w344) -> ("Decimated and Filtered Array"=w345:dbl[])  [unwired: 6 in, 1 out]
            n128 = Bundle By Name(cluster=w344, "Y"=w345) -> (w343:waveform(dbl))
          }
          n129 = for {
            tunnel: "low cutoff freq: fl" -> [w353]
            tunnel: w341 -> [w350] mode=indexing
            tunnel: "decimating factor" -> [w354]
            tunnel: "Enable Filter?" -> [w352]
            tunnel: [w349] -> w333 mode=indexing
            n130 = call "Decimate and Filter.vi"("Enabled?"=w352, "low cutoff freq: fl"=w353, "decimating factor"=w354, "Waveform in"=w350) -> ("Decimated and Filtered Array"=w351:dbl[])  [unwired: 6 in, 1 out]
            n131 = Bundle By Name(cluster=w350, "Y"=w351) -> (w349:waveform(dbl))
          }
          n132 = Bundle By Name(cluster=w334, "AI"=w333, "AO"=w332) -> (w331:T15)
        }
        n133 = Bundle By Name(cluster=w326, "IVSweepResults (filtered).IVSweepResults []"=w324) -> (w325:T10)
        n134 = call <vilib>:"Add State(s) to Queue__jki_lib_state_machine.vi"("State(s) in (\"\")"=w330) -> ("States Out"=w329:string)  [unwired: 14 in]
      }
      frame "---------- File ----------" {
        # "Do not put any code in this frame.\n(It is a separator no-op. You can make a copy of this frame to create a new Macro frame)"
        n135 = call <vilib>:"Add State(s) to Queue__jki_lib_state_machine.vi"("State(s) in (\"\")"=w363) -> ("States Out"=w362:string)  [unwired: 14 in]
      }
      frame "File: Save" {
        # "Do not put any code in this frame.\n(It is a separator no-op. You can make a copy of this frame to create a new Macro frame)"
        n136 = Unbundle By Name(w375) -> ("Control Experiment"=w371:refnum<class "Control Experiment.lvclass">, "Temperature"=w374:dbl, "Magnet"=w373:dbl, "IVSweepResults (filtered).IVSweepResults []"=w372:T14)
        n137 = call <userlib>:"Tick Count (ms)__ogtk.vi"("error in (no error)"=w370) -> ("error out"=w368:errorcluster, "millisecond timer value"=w365:u32)  [unwired: 9 in]
        n138 = for {
          tunnel: w374 -> [w401]
          tunnel: w373 -> [w400]
          tunnel: w372 -> [w398] mode=indexing
          tunnel: w371 -> [w391]
          shift-right: [w379] -> w369
          shift-left: w368 -> [w388]
          n139 = Unbundle By Name(w398) -> ("AI"=w384:waveform(dbl)[], "AO"=w383:waveform(dbl)[])
          n140 = Build Array(w400) -> (w399:dbl[])
          n141 = Build Array(w401) -> (w396:dbl[])
          n142 = for {
            tunnel: w383 -> [w404] mode=indexing
            tunnel: [w402] -> w393 mode=indexing
            n143 = Unbundle By Name(w404) -> ("Y"=w403:dbl[])
            n144 = Bundle("Y"=w403) -> (w402:cluster{"Y":dbl[]})  [unwired: 1 in]
          }
          n145 = for {
            tunnel: w384 -> [w407] mode=indexing
            tunnel: [w405] -> w392 mode=indexing
            n146 = Unbundle By Name(w407) -> ("Y"=w406:dbl[])
            n147 = Bundle("Y"=w406) -> (w405:cluster{"Y":dbl[]})  [unwired: 1 in]
          }
          n148 = Array Size(array=w384) -> (size(s)=w386:i32)
          n149 = Array Size(array=w383) -> (size(s)=w387:i32)
          n150 = call "Create Keys (AI).vi"("Numeric"=w386) -> ("AI Keys"=w385:string[])  [unwired: 2 in]
          n151 = call "Create Keys (AO).vi"("Numeric"=w387) -> ("AO Keys"=w382:string[])  [unwired: 2 in]
          n152 = Build Cluster Array(dbl[] [1.0] ("element"), w396, w399) -> (w397:cluster{"element":dbl[]}[])
          n153 = Build Array (concatenate)(w397, w392, w393) -> (w389:cluster{"Y":dbl[]}[])
          n154 = Build Array (concatenate)(string[] ["time", "temp", "B"] ("wavenames (.Vx, etc)"), w385, w382) -> (w390:string[])
          n155 = call "Write Dictionary Elements (Loop).vi"("error in (no error)"=w388, "values"=w389, "keys"=w390, "Control Experiment in"=w391) -> ("error out"=w380:errorcluster, "Control Experiment out"=w381:refnum<class "Control Experiment.lvclass">)  [unwired: 6 in]
          n156 = call "Save Transport TDMS File.vi"("error in (no error)"=w380, "append?"=TRUE, "Control Experiment in"=w381) -> ("error out"=w379:errorcluster)  [unwired: 7 in, 1 out]
        }
        n157 = call <userlib>:"Tick Count (ms)__ogtk.vi"("error in (no error)"=w369) -> ("error out"=w367:errorcluster, "millisecond timer value"=w366:u32)  [unwired: 9 in]
        n158 = call <vilib>:"Add State(s) to Queue__jki_lib_state_machine.vi"("State(s) in (\"\")"=w377) -> ("States Out"=w376:string)  [unwired: 14 in]
        n159 = Subtract(x=w366, y=w365) -> (x-y=→"time to write files (ms)":u32)
      }
    }
  }
  n160 = Unbundle By Name(w9) -> ("Transport"=→"Transport out":refnum<class "Transport.lvclass">)
  n161 = call <userlib>:"Tick Count (ms)__ogtk.vi"("error in (no error)"=w6) -> ("error out"=→"error out":errorcluster, "millisecond timer value"=w3:u32)  [unwired: 9 in]
  n162 = Subtract(x=w3, y=w2) -> (x-y=→"total time (ms)":u32)
